vi "Fetch Multi Eval Meas Power Monitor Results.vi"(8 "error in (no error)":errorcluster, 9 "Result Type (Current)":i32(ring) items=["Current"=0, "Average"=1, "Standard Deviation"=3, "Maximum"=4, "Minimum"=5], 10 "Instance (1)":T1=1, 11 "VISA resource name":refnum<visa-resource-name>) -> (0 "error out":errorcluster, 1 "Out Of Tolerance":i32, 2 "Reliability":i32, 3 "VISA resource name out":refnum<visa-resource-name>, 4 "Total TX Power":dbl format="%^.3e")   [LabVIEW 2020, in "Rohde&Schwarz CMWXP NR FR1 Measurement.lvlib"]
doc: "Returns the total TX power. The current, average, standard deviation, maximum, and minimum results can be returned.\n\nAttributes:\nRSCMWXPNRFR1M_ATTR_FETCH_MULTI_EVAL_MEAS_POWER_MONITOR_CURRENT_RESULTS\nRSCMWXPNRFR1M_ATTR_FETCH_MULTI_EVAL_MEAS_POWER_MONITOR_AVERAGE_RESULTS\nRSCMWXPNRFR1M_ATTR_FETCH_MULTI_EVAL_MEAS_POWER_MONITOR_STANDARD_DEVIATION_RESULTS\nRSCMWXPNRFR1M_ATTR_FETCH_MULTI_EVAL_MEAS_POWER_MONITOR_MAXIMUM_RESULTS\nRSCMWXPNRFR1M_ATTR_FETCH_MULTI_EVAL_MEAS_POWER_MONITOR_MINIMUM_RESULTS\n\nRemote-control commands:\nFETCh:NRSub:MEAS<i>:MEValuation:PMONitor:CURRent?\nFETCh:NRSub:MEAS<i>:MEValuation:PMONitor:AVERage?\nFETCh:NRSub:MEAS<i>:MEValuation:PMONitor:SDEViation?\nFETCh:NRSub:MEAS<i>:MEValuation:PMONitor:MAXimum?\nFETCh:NRSub:MEAS<i>:MEValuation:PMONitor:MINimum?"
uses:
  <instrlib>/Rohde&Schwarz CMWXP NR FR1 Measurement/Rohde&Schwarz CMWXP NR FR1 Measurement.lvlib
  <instrlib>/Rohde&Schwarz CMWXP NR FR1 Measurement/Private/_Instance.ctl
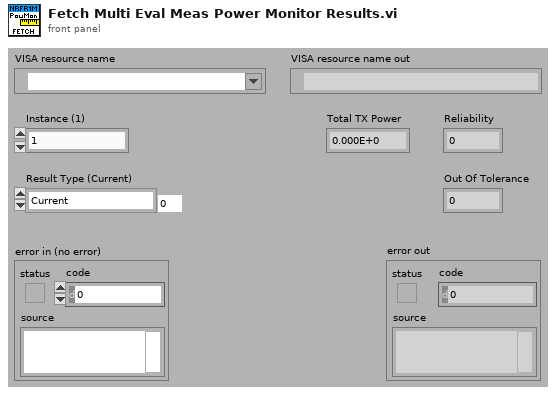
[diagram p1: front panel]
types:
  T1 = typedef "Rohde&Schwarz CMWXP NR FR1 Measurement.lvlib/_Instance.ctl" = i32
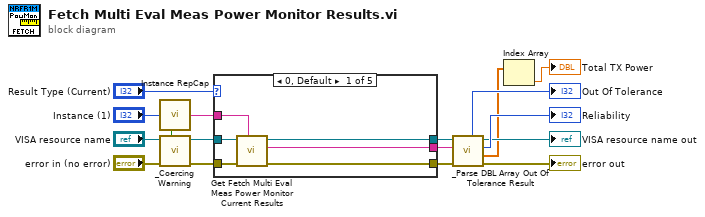
[diagram p0: block diagram]
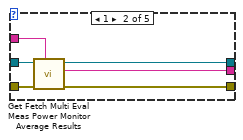
[diagram p2: hidden frame]
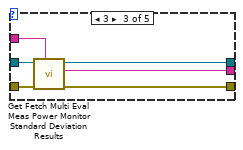
[diagram p3: hidden frame]
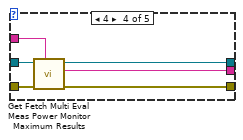
[diagram p4: hidden frame]
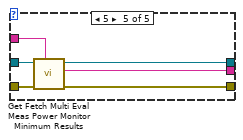
[diagram p5: hidden frame]
diagram:
  n1 = call <instrlib>:"Instance RepCap.vi"("Instance In"="Instance (1)") -> ("In Range?"=w14:bool, "RepCap Identifier Out"=w13:string)  [unwired: 1 in]
  n2 = call <instrlib>:"_Coercing Warning.vi"("In Range?"=w14, "error in (no error)"="error in (no error)", "VISA resource name"="VISA resource name") -> ("error out"=w11:errorcluster, "VISA resource name out"=w12:refnum<visa-resource-name>)  [unwired: 7 in]
  n3 = case shown="0, Default" "Result Type (Current)" {
    tunnel: w13 -> [w23 w29 w35 w41 w47]
    tunnel: w12 -> [w22 w28 w34 w40 w46]
    tunnel: w11 -> [w21 w27 w33 w39 w45]
    tunnel: [w20 w26 w32 w38 w44] -> w7
    tunnel: [w19 w25 w31 w37 w43] -> w8
    tunnel: [w18 w24 w30 w36 w42] -> w9
    frame 0, Default {
      n4 = call "Get Fetch Multi Eval Meas Power Monitor Current Results"("Repeated Capabilities"=w23, "error in (no error)"=w21, "instrument handle"=w22) -> ("error out"=w18:errorcluster, "Fetch Multi Eval Meas Power Monitor Current Results"=w19:string, "instrument handle out"=w20:refnum<visa-resource-name>)  [unwired: 6 in]
    }
    frame 1 {
      n5 = call "Get Fetch Multi Eval Meas Power Monitor Average Results"("Repeated Capabilities"=w29, "error in (no error)"=w27, "instrument handle"=w28) -> ("error out"=w24:errorcluster, "Fetch Multi Eval Meas Power Monitor Average Results"=w25:string, "instrument handle out"=w26:refnum<visa-resource-name>)  [unwired: 6 in]
    }
    frame 3 {
      n6 = call "Get Fetch Multi Eval Meas Power Monitor Standard Deviation Results"("Repeated Capabilities"=w35, "error in (no error)"=w33, "instrument handle"=w34) -> ("error out"=w30:errorcluster, "Fetch Multi Eval Meas Power Monitor Standard Deviation Results"=w31:string, "instrument handle out"=w32:refnum<visa-resource-name>)  [unwired: 6 in]
    }
    frame 4 {
      n7 = call "Get Fetch Multi Eval Meas Power Monitor Maximum Results"("Repeated Capabilities"=w41, "error in (no error)"=w39, "instrument handle"=w40) -> ("error out"=w36:errorcluster, "Fetch Multi Eval Meas Power Monitor Maximum Results"=w37:string, "instrument handle out"=w38:refnum<visa-resource-name>)  [unwired: 6 in]
    }
    frame 5 {
      n8 = call "Get Fetch Multi Eval Meas Power Monitor Minimum Results"("Repeated Capabilities"=w47, "error in (no error)"=w45, "instrument handle"=w46) -> ("error out"=w42:errorcluster, "Fetch Multi Eval Meas Power Monitor Minimum Results"=w43:string, "instrument handle out"=w44:refnum<visa-resource-name>)  [unwired: 6 in]
    }
  }
  n9 = call <instrlib>:"_Parse DBL Array Out Of Tolerance Result.vi"("error in (no error)"=w9, "Input String"=w8, "VISA resource name"=w7) -> ("error out"=→"error out":errorcluster, "Results"=w2:dbl[], "Reliability"=→"Reliability":i32, "VISA resource name out"=→"VISA resource name out":refnum<visa-resource-name>, "Out Of Tolerance"=→"Out Of Tolerance":i32)  [unwired: 4 in]
  n10 = Index Array(array=w2) -> (element=→"Total TX Power":dbl)  [unwired: 1 in]
